vi "A 侧面 处理函数CCD3.vi"(8 "error in (no error)":errorcluster caption="错误输入（无错误）", 9 "相机选择":T2="CCD4" caption="Session Out CCD3", 10 "New Image":T1, 11 "ParamsUI":T3={"IsNorImage"=TRUE, "Exposure Values"=100289, "ImagePath"=path "C:/Users/hedongpo/Desktop/514-hdp/Alignment Assemble System/Test Picture/B/3.bmp", "相机选择"="cam4"} caption="参数界面" {"Exposure Values" scale=0.0..200000.0}) -> (0 "error out":errorcluster caption="错误输出", 2 "Session Out":T2, 3 "Image out":T1(plugin-control), 4 "数值":dbl)   [LabVIEW 2017]
uses:
  <vilib>/userdefined/High Color/IMAQdx.ctl
  <vilib>/vision/Image Controls.llb/IMAQ Image.ctl
  <vilib>/vision/driver/IMAQdx.llb/IMAQdx Buffer Number Mode.ctl
  <resource>/objmgr/imaqdx.rc
  Global System.vi
  <vilib>/vision/driver/NI_Vision_Acquisition_Software.lvlib
  <vilib>/vision/NI_Vision_Development_Module.lvlib
panel:
  in  "Image Name":string="I123"
  in  "相机选择":string(combo)
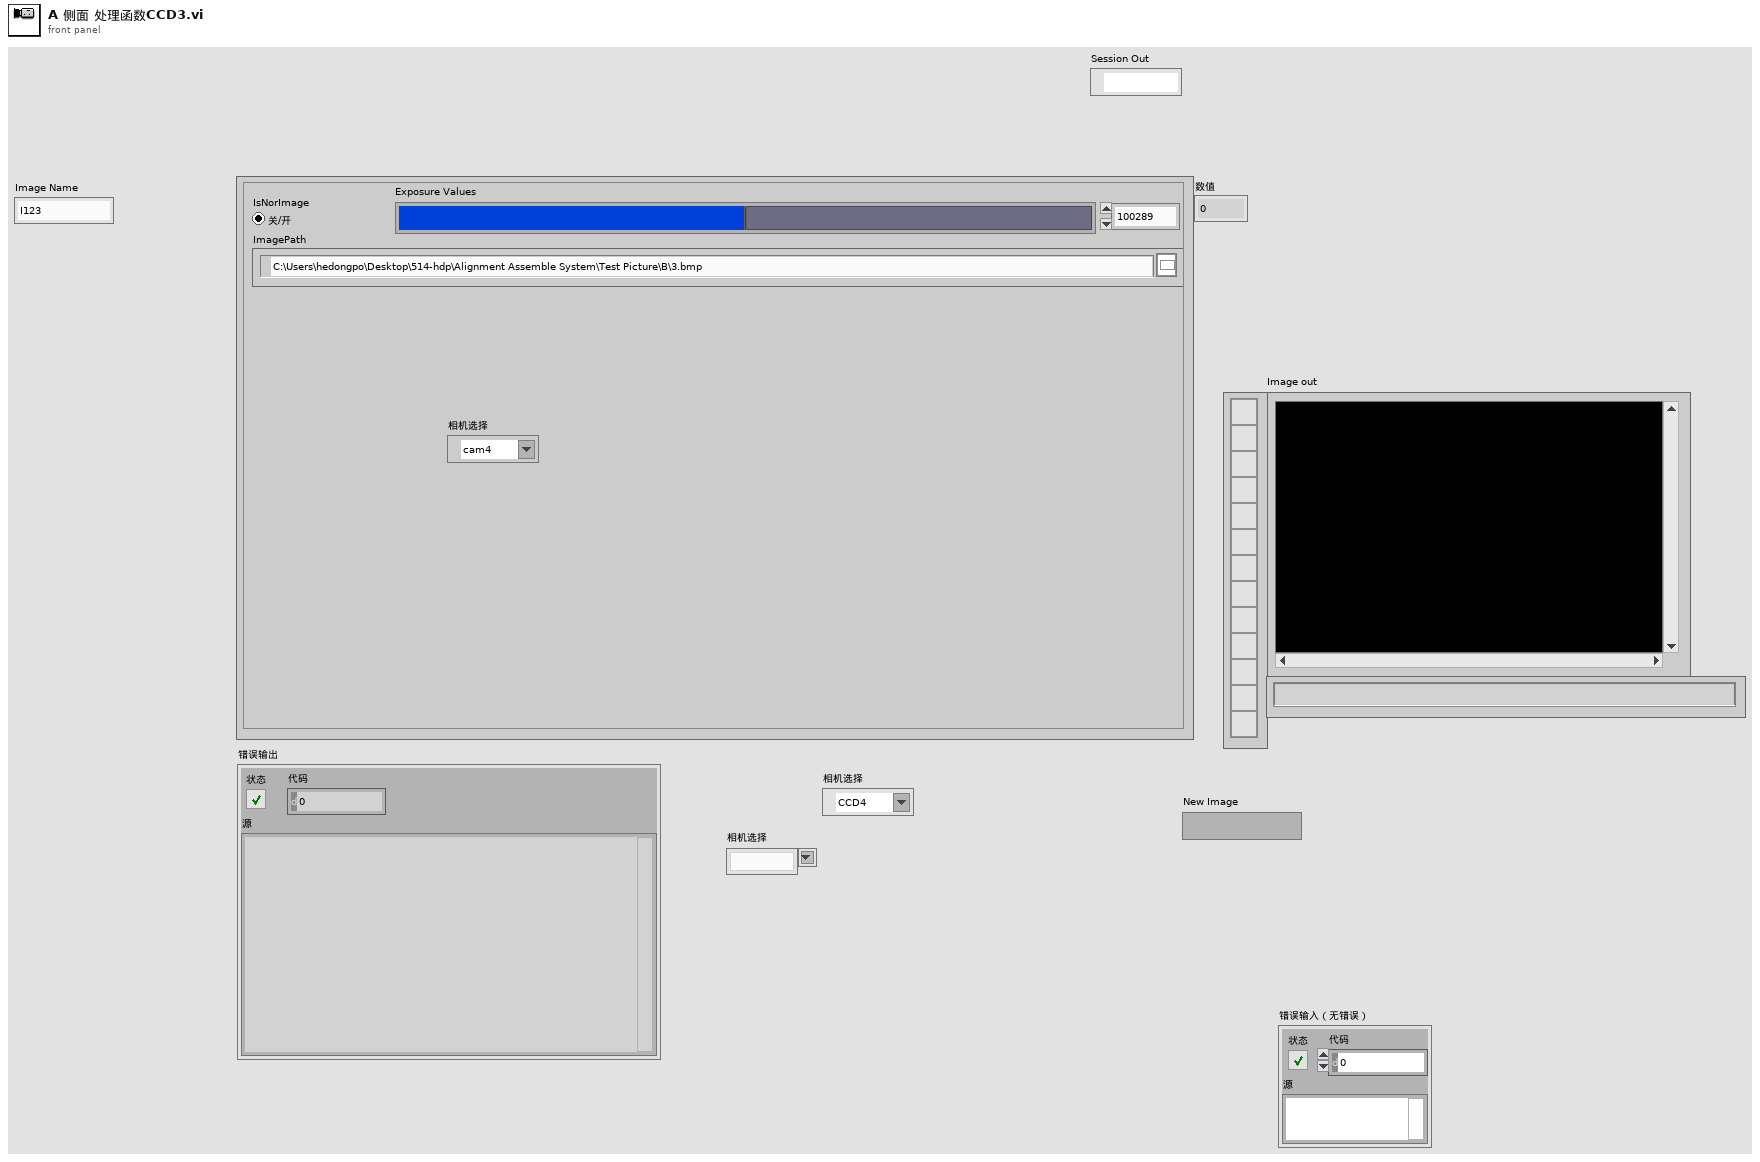
[diagram p1: front panel]
types:
  T1 = typedef "IMAQ Image.ctl" = refnum<image>
  T2 = typedef "IMAQdx.ctl" = refnum<k21>
  T3 = cluster{"IsNorImage":bool, "Exposure Values":i64, "ImagePath":path, "相机选择":T2}
  T4 = typedef "Image Type" = u32
  T5 = cluster{"IsNorImage":bool, "Exposure Values":u32, "ImagePath":path}
  T6 = typedef "NI_Vision_Acquisition_Software.lvlib/IMAQdx Buffer Number Mode.ctl" = enum32{"Next", "Last", "Buffer Number", "Every", "Last New"}
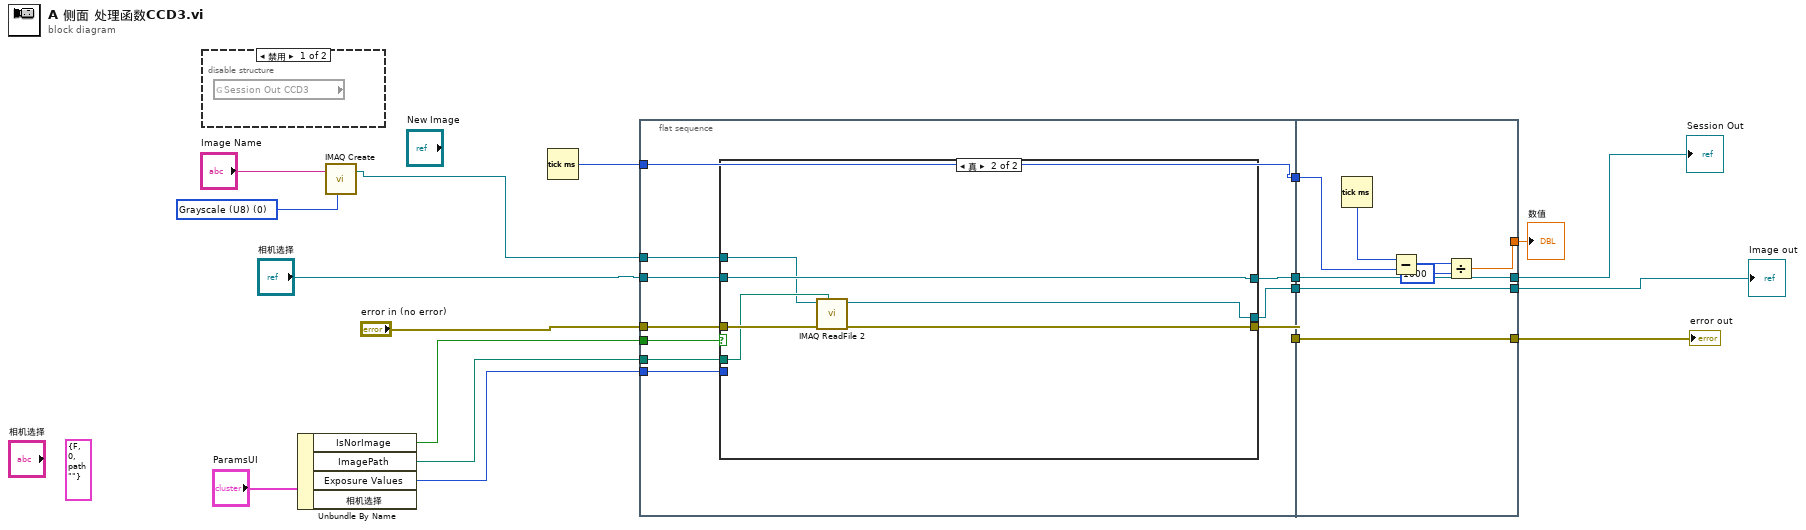
[diagram p0: block diagram]
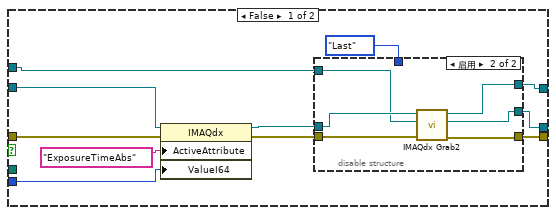
[diagram p3: hidden frame]
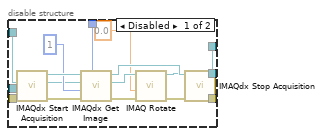
[diagram p4: hidden frame]
diagram:
  w2 = T4 0 items=["Grayscale (U8)", "Grayscale (I16)", "Grayscale (SGL)", "Complex (CSG)", "RGB (U32)", "HSL (U32)", "RGB (U64)", "Grayscale (U16)"] ("Image Type")
  (unwired) T5 {"IsNorImage"=FALSE, "Exposure Values"=0, "ImagePath"=path ""} ("ParamsUI")
  n1 = disable-structure shown="禁用" {
    frame Disabled {
      n2 = global read "Global System.vi" "Session Out CCD3"() -> ()  [unwired: 1 out]
    }
    frame Enabled {
    }
  }
  n3 = Unbundle By Name("ParamsUI") -> ("IsNorImage"=w5:bool, "ImagePath"=w6:path, "Exposure Values"=w18:i64)  [unwired: 1 out]
  n4 = call "IMAQ Create"("Image Name"="Image Name", "Image Type"=w2) -> ("New Image"=w1:T1)  [unwired: 3 in, 1 out]
  n5 = Tick Count (ms)() -> (millisecond timer value=w12:u32)
  n6 = flat-sequence {
    tunnel: w5 -> [w28]
    tunnel: w6 -> [w27]
    tunnel: w18 -> [w26]
    tunnel: w1 -> [w25]
    tunnel: "error in (no error)" -> [w24]
    tunnel: "相机选择" -> [w21]
    tunnel: w12 -> [w19]
    tunnel: [w23] -> w11
    tunnel: [w22] -> w10
    tunnel: [w20] -> w9
    tunnel: [w19] -> w8
    tunnel: [w67] -> w13
    tunnel: [w73] -> w14
    tunnel: [w74] -> w16
    tunnel: w11 -> [w74]
    tunnel: w10 -> [w73]
    tunnel: w9 -> [w67]
    tunnel: w8 -> [w71]
    tunnel: [w68] -> w7
    frame #0 {
      n7 = case shown="真" w28 {
        tunnel: w27 -> [_ w62]
        tunnel: [w37 w63] -> w22
        tunnel: w26 -> [w32 _]
        tunnel: w21 -> [w34 w66]
        tunnel: w25 -> [w38 w61]
        tunnel: w24 -> [w33 w65]
        tunnel: [w35 w64] -> w23
        tunnel: [w36 w66] -> w20
        frame False {
          n8 = property class="IMAQdx"(reference=w34, error in=w33, "ActiveAttribute"="ExposureTimeAbs", "ValueI64"=w32) -> (reference out=w31:T2, error out=w30:errorcluster)
          n9 = disable-structure shown="启用" {
            disable-tunnel: IMAQdx_Buffer_Number_Mode."Last" ("Buffer Number Mode (Next)") -> [w51 _]
            disable-tunnel: w38 -> [w45 w56]
            disable-tunnel: [w44 w55] -> w37
            disable-tunnel: [w43 w57] -> w36
            disable-tunnel: [w42 w58] -> w35
            disable-tunnel: w31 -> [w41 w60]
            disable-tunnel: w30 -> [w40 w59]
            frame Disabled {
              n10 = call <vilib>:"IMAQdx Start Acquisition.vi"("error in"=w40, "Session In"=w41) -> ("error out"=w53:errorcluster, "Session Out"=w54:T2)  [unwired: 8 in]
              n11 = call <vilib>:"IMAQdx Get Image.vi"("Buffer Number Mode (Next)"=w51, "error in"=w53, "Buffer Number In"=u32 1, "Image In"=w45, "Session In"=w54) -> ("error out"=w48:errorcluster, "Image Out"=w49:T1, "Session Out"=w50:T2)  [unwired: 3 in, 1 out]
              n12 = call "IMAQ Rotate"("error in (no error)"=w48, "Angle (degrees)"=sgl 0.0, "Image Src"=w49) -> ("error out"=w47:errorcluster, "Image Dst Out"=w44:T1)  [unwired: 7 in]
              n13 = call <vilib>:"IMAQdx Stop Acquisition.vi"("error in"=w47, "Session In"=w50) -> ("error out"=w42:errorcluster, "Session Out"=w43:T2)  [unwired: 8 in]
            }
            frame Enabled {
              n14 = call <vilib>:"IMAQdx Grab2.vi"("error in"=w59, "Image In"=w56, "Session In"=w60) -> ("error out"=w58:errorcluster, "Image Out"=w55:T1, "Session Out"=w57:T2)  [unwired: 5 in, 1 out]
            }
          }
        }
        frame True {
          n15 = call "IMAQ ReadFile 2"("File Path"=w62, "error in (no error)"=w65, "Image"=w61) -> ("error out"=w64:errorcluster, "Image Out"=w63:T1)  [unwired: 4 in, 3 out]
        }
      }
    }
    frame #1 {
      n16 = Tick Count (ms)() -> (millisecond timer value=w72:u32)
      n17 = Subtract(x=w72, y=w71) -> (x-y=w70:u32)
      n18 = Divide(x=w70, y=u32 1000) -> (x/y=w68:dbl)
    }
  }
  "Image out" <- w14
  "error out" <- w16
  "Session Out" <- w13
  "数值" <- w7
